vi "Stop Simulation.vi"() -> ()   [LabVIEW 2018]
doc: "Imports MAX Configuration from specified location."
uses:
  <vilib>/Utility/error.llb/DialogType.ctl
  <vilib>/nisyscfg/Close (System).vi
  <vilib>/nisyscfg/nisyscfg.lvlib
  <resource>/objmgr/nisysapi.rc
panel:
  in  "User Name":string
  in  "Password":string
  in  "Target (localhost)":refnum<k21>="localhost"
  # "Overview: Imports MAX Configuration from a specified location.\nRequirements: NI System Configuration, NI MAX\nInstructions:\n1. Select Target. Enter User Name and Password if necessary.\n2. Specify the location of the configuration file in File Path. \n3. Run the VI."
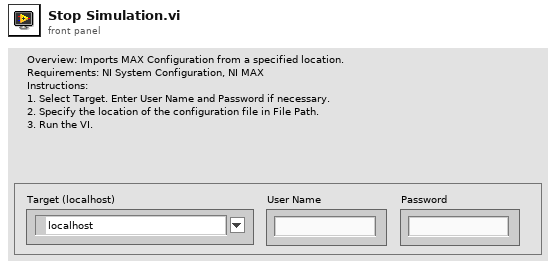
[diagram p1: front panel]
types:
  T1 = typedef "DialogType.ctl" = u16
  T2 = enum32{"invalid app kind", "Development System", "Run Time System", "Student Edition", "Embedded LabVIEW", "Evaluation", "Custom"}
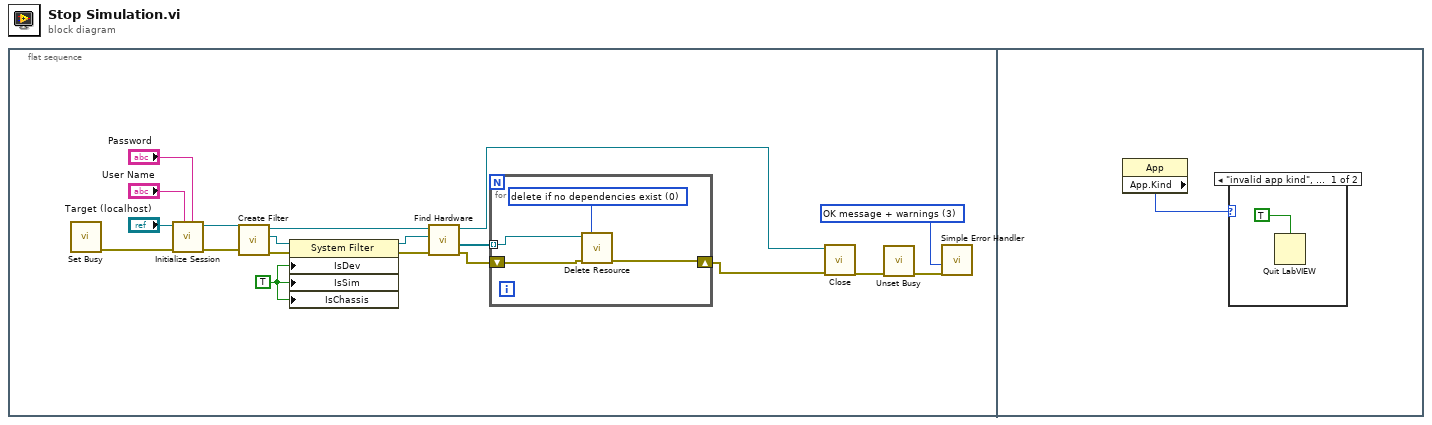
[diagram p0: block diagram]
diagram:
  n1 = flat-sequence {
    frame #0 {
      w3 = TRUE ("Is Chassis")
      w17 = T1 3 items=["no dialog", "OK message", "continue or stop message", "OK message + warnings", "continue/stop + warnings"] ("type of dialog (OK msg:1)")
      n2 = call <vilib>:"Set Busy.vi"() -> ("error out"=w13:errorcluster)  [unwired: 10 in, 1 out]
      n3 = call <vilib>:"Initialize Session.vi"("Password"="Password", "User Name"="User Name", "error in (no error)"=w13, "Target (localhost)"="Target (localhost)") -> ("error out"=w1:errorcluster, "Session out"=w2:refnum<k21>)  [unwired: 6 in]
      n4 = call <vilib>:"Create Filter.vi"("error in (no error)"=w1, "Session in"=w2) -> ("error out"=w12:errorcluster, "Filter out"=w11:refnum<k20>, "Session out"=w10:refnum<k21>)  [unwired: 7 in]
      n5 = property class="System Filter"(reference=w11, error in=w12, "IsDev"=w3, "IsSim"=w3, "IsChassis"=w3) -> (reference out=w8:refnum<k20>, error out=w9:errorcluster)
      n6 = call <vilib>:"Find Hardware.vi"("error in (no error)"=w9, "Filter in"=w8, "Session in"=w10) -> ("error out"=w6:errorcluster, "Resources out"=w7:refnum<k20>[], "Session out"=w4:refnum<k21>)  [unwired: 1 in, 5 out]
      n7 = for {
        tunnel: w7 -> [w23] mode=indexing
        shift-right: [w21] -> w5
        shift-left: w6 -> [w22]
        w20 = 0 items=["validate but do not delete"=-1, "delete if no dependencies exist"=0, "delete item and any dependencies"=1, "delete item but keep dependencies"=2] ("Delete Mode")
        n8 = call <vilib>:"Delete Resource.vi"("error in (no error)"=w22, "Delete Mode"=w20, "Resource in"=w23) -> ("error out"=w21:errorcluster)  [unwired: 5 in, 3 out]
      }
      n9 = call-poly <vilib>:"Close.vi"("error in (no error)"=w5, "Session in"=w4) -> ("error out"=w19:errorcluster)  [unwired: 9 in]
      n10 = call <vilib>:"Unset Busy.vi"("error in (no error)"=w19) -> ("error out"=w18:errorcluster)  [unwired: 10 in]
      n11 = call <vilib>:"Simple Error Handler.vi"("type of dialog (OK msg:1)"=w17, "error in (no error)"=w18) -> ()  [unwired: 3 in, 5 out]
    }
    frame #1 {
      n12 = property class="App"() -> ("App.Kind"=w24:T2)  [unwired: 2 in, 2 out]
      n13 = case shown="\"invalid app kind\", Default" w24 {
        frame "invalid app kind", Default {
          n14 = Quit LabVIEW(quit? (T)=TRUE) -> ()
        }
        frame "Development System" {
        }
      }
    }
  }
